vi "Data Manager.vi"(8 "error in (no error)":errorcluster, 9 "Mode":enum16{"Store Data", "Get Data", "Cleanup"}(ring)=enum."Get Data", 10 "Data In":T1 {"Serial Communication"."Baud Rate" items=["75"=75, "110"=110, "134"=134, "150"=150, "300"=300, "600"=600, "1200"=1200, "1800"=1800, "2400"=2400, "4800"=4800, "7200"=7200, "9600"=9600, "14400"=14400, "19200"=19200, "28800"=28800, "38400"=38400, "56000"=56000, "57600"=57600, "115200"=115200, "128000"=128000, "230400"=230400]}, 11 "Refnum In":refnum<vi>) -> (0 "error out":errorcluster, 2 "Data Out":T1={"Serial Communication"={"Comport"="", "No Response Timeout Ms"=5000, "Response Complete Timeout Ms"=200, "Max Rx Length"=1048, "Baud Rate"=9600}, "Selected Transport"=enum."Serial Communication Port", "Initializer File Path"=path "", "Cleaner File Path"=path "", "Transporter File Path"=path ""} {"Serial Communication"."Baud Rate" items=["75"=75, "110"=110, "134"=134, "150"=150, "300"=300, "600"=600, "1200"=1200, "1800"=1800, "2400"=2400, "4800"=4800, "7200"=7200, "9600"=9600, "14400"=14400, "19200"=19200, "28800"=28800, "38400"=38400, "56000"=56000, "57600"=57600, "115200"=115200, "128000"=128000, "230400"=230400]}, 3 "Refnum Out":refnum<vi>)   [LabVIEW 2020]
uses:
  Controls/ConnectionParameters.ctl
  Controls/SupportedTransports.ctl
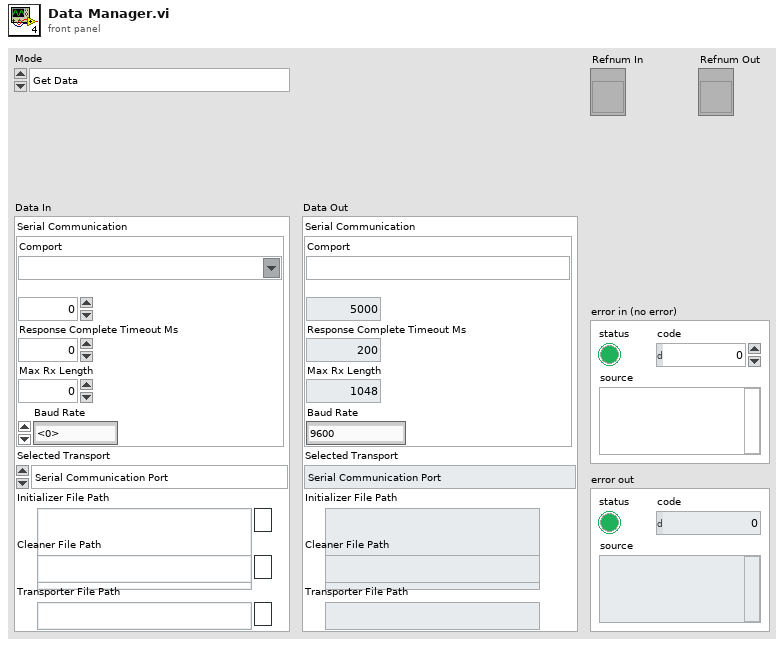
[diagram p1: front panel]
types:
  T1 = typedef "ConnectionParameters.ctl" = cluster{"Serial Communication":cluster{"Comport":refnum<visa-resource-name>, "No Response Timeout Ms":u32, "Response Complete Timeout Ms":u32, "Max Rx Length":u32, "Baud Rate":u32}, "Selected Transport":T2, "Initializer File Path":path, "Cleaner File Path":path, "Transporter File Path":path}
  T2 = typedef "SupportedTransports.ctl" = enum16{"Serial Communication Port"}
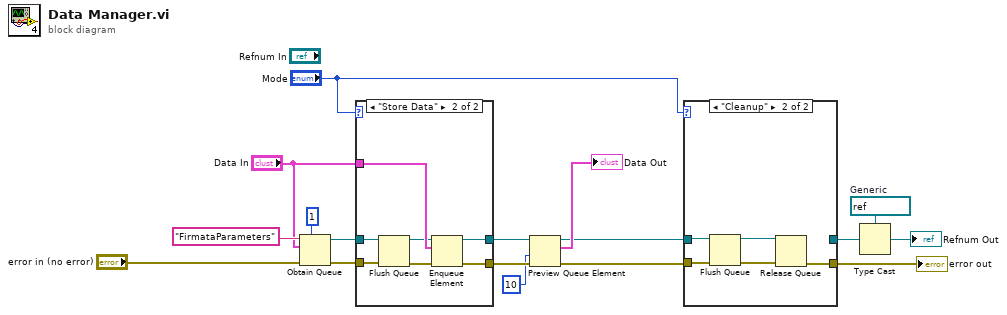
[diagram p0: block diagram]
diagram:
  w14 = refnum<vi> refnum  # Generic
  n1 = Obtain Queue(max queue size (-1, unlimited)=1, name (unnamed)="FirmataParameters", element data type="Data In", error in (no error)="error in (no error)") -> (queue out=w12:refnum<queue>, error out=w16:errorcluster)  [unwired: 1 in, 1 out]
  n2 = case shown="\"Store Data\"" "Mode" {
    tunnel: w16 -> [w18 w22]
    tunnel: "Data In" -> [_ w26]
    tunnel: w12 -> [w19 w23]
    tunnel: [w18 w25] -> w10
    tunnel: [w19 w24] -> w9
    frame Default {
    }
    frame "Store Data" {
      n3 = Flush Queue(queue=w23, error in (no error)=w22) -> (queue out=w21:refnum<queue>, error out=w20:errorcluster)  [unwired: 1 out]
      n4 = Enqueue Element(queue=w21, element=w26, error in (no error)=w20) -> (queue out=w24:refnum<queue>, error out=w25:errorcluster)  [unwired: 1 in, 1 out]
    }
  }
  n5 = Preview Queue Element(queue=w9, timeout in ms (-1)=10, error in (no error)=w10) -> (queue out=w7:refnum<queue>, element=→"Data Out":T1, error out=w6:errorcluster)  [unwired: 1 out]
  n6 = case shown="\"Cleanup\"" "Mode" {
    tunnel: w6 -> [w27 w32]
    tunnel: w7 -> [w28 w30]
    tunnel: [w27 w33] -> w5
    tunnel: [w28 _] -> w4
    frame Default {
    }
    frame "Cleanup" {
      n7 = Flush Queue(queue=w30, error in (no error)=w32) -> (queue out=w29:refnum<queue>, error out=w31:errorcluster)  [unwired: 1 out]
      n8 = Release Queue(queue=w29, error in (no error)=w31) -> (error out=w33:errorcluster)  [unwired: 1 in, 2 out]
    }
  }
  "error out" <- w5
  n9 = Type Cast(type=w14, x=w4) -> (*(type *) &x=→"Refnum Out":refnum<vi>)
